vi "Signal.vi"() -> ()   [LabVIEW 2023]
doc: "Use this template to simulate the generation and display of data.\nNote: LabVIEW enables automatic error handling by default for VIs you create from this template."
uses:
  Instance           1 27Saved   GenerateDisplay.vit .vi
panel:
  in  "Knob":dbl(knob) scale=0.0..10.0
  out "Waveform Graph":dynamicdata(graph)
  in  "stop":bool
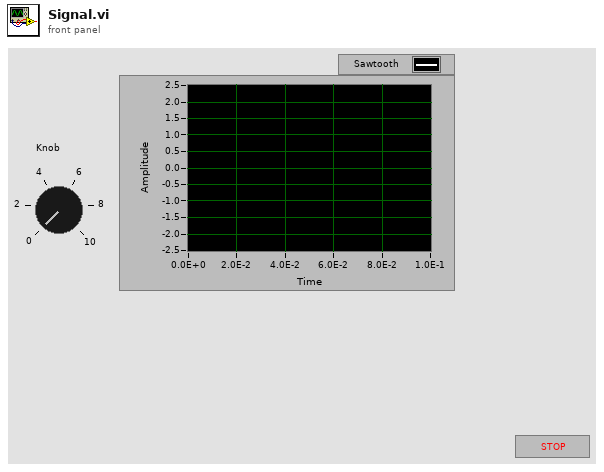
[diagram p1: front panel]
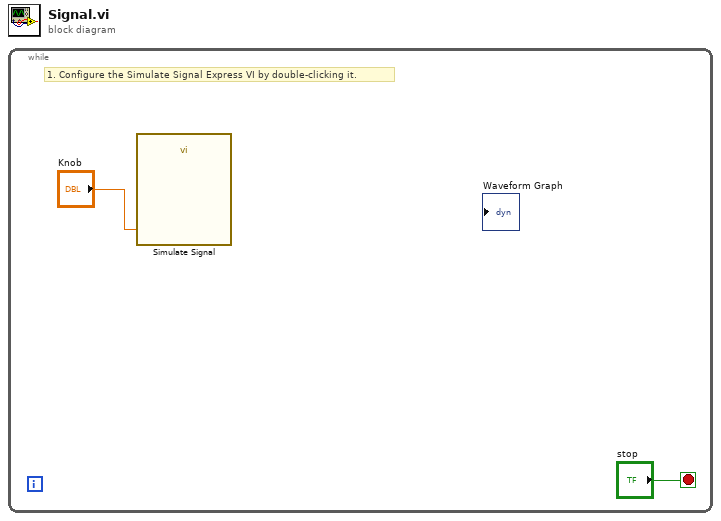
[diagram p0: block diagram]
diagram:
  n1 = while {
    stop <- "stop" stop-if-true
    # "1. Configure the Simulate Signal Express VI by double-clicking it."
    n2 = call "Simulate Signal"("Amplitude"="Knob") -> ()  [unwired: 13 in, 2 out]
  }
